vi "string pattern counter.vi"(9 "pattern":string="root", 11 "string":string="root\nroot\nroot\nroot") -> (2 "Numeric":i32)   [LabVIEW 2021]
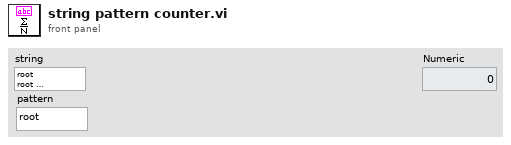
[diagram p1: front panel]
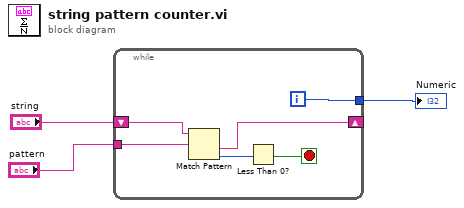
[diagram p0: block diagram]
diagram:
  n1 = while {
    tunnel: [w5] -> w3
    shift-right: [w7] -> _
    shift-left: "string" -> [w6]
    tunnel: "pattern" -> [w4]
    i -> [w5]
    stop <- w8 stop-if-true
    n2 = Match Pattern(string=w6, regular expression=w4) -> (after substring=w7:string, offset past match=w9:i32)  [unwired: 1 in, 2 out]
    n3 = Less Than 0?(x=w9) -> (x < 0?=w8:bool)
  }
  "Numeric" <- w3
